vi "MoveOneRow.vi"(2 "#ofMoveRows":i32, 3 "Table In Ref":refnum<vi>, 5 "Table In":string[][](array[string])) -> (1 "Table Out":string[][](array[string]))   [LabVIEW 2012]
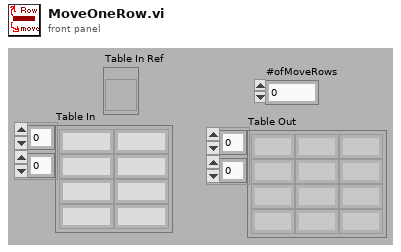
[diagram p1: front panel]
types:
  T1 = typedef "LVRowAndColumnTypeDef.ctl" = cluster{"Row":i32, "Column":i32}
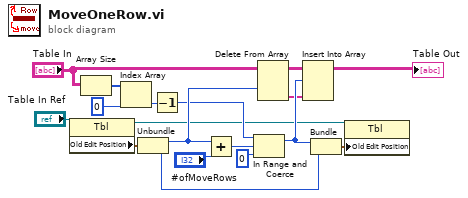
[diagram p0: block diagram]
diagram:
  n1 = property class="Tbl"(reference="Table In Ref") -> (reference out=w7:refnum<vi>, "Old Edit Position"=w2:T1)  [unwired: 1 in, 1 out]
  n2 = Array Size(array="Table In") -> (size(s)=w10:i32[])
  n3 = Index Array(array=w10, index=0) -> (element=w12:i32)
  n4 = Unbundle(w2) -> ("Row"=w16:i32, "Column"=w8:i32)
  n5 = Decrement(x=w12) -> (x-1=w13:i32)
  n6 = Add(x=w16, y="#ofMoveRows") -> (x+y=w17:i32)
  n7 = In Range and Coerce(upper limit=w13, x=w17, lower limit=0) -> (coerced(x)=w15:i32)  [unwired: 1 out]
  n8 = Delete From Array(array="Table In", index (row)=w16) -> (deleted portion=w3:string[], array with subset deleted=w1:string[][])  [unwired: 2 in]
  n9 = Insert Into Array(array=w1, index (row)=w15, new element=w3) -> (→"Table Out":string[][])  [unwired: 1 in]
  n10 = Bundle("lower limit"=w15, "Column"=w8) -> (w6:cluster{"lower limit":i32, "Column":i32})  [unwired: 1 in]
  n11 = property class="Tbl"(reference=w7, "Old Edit Position"=w6) -> ()  [unwired: 1 in, 2 out]
